vi "Add Parent.vi"(8 "error in (no error)":errorcluster, 9 "Parent ID":i32=-1, 10 "Object ID":i32=-1, 11 "Parent Child in":refnum<class "Parent Child.lvclass">) -> (0 "error out":errorcluster, 3 "Parent Child out":refnum<class "Parent Child.lvclass">)   [LabVIEW 2019, in "HierDAL Library.lvlib" / "Database.lvlib" / "Repositories.lvlib" / "Parent Child.lvclass"]
uses:
  Parent Child.lvclass
  Parent Child.lvclass/Parent Child.ctl
  Database Manager Class/Database Manager.lvclass
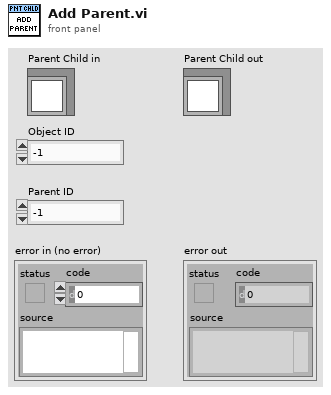
[diagram p1: front panel]
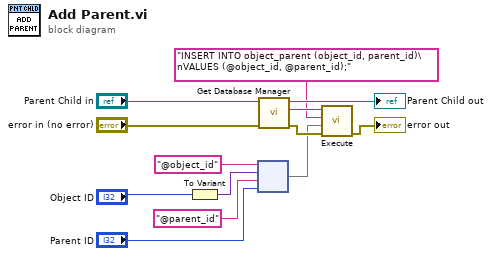
[diagram p0: block diagram]
diagram:
  n1 = To Variant(anything="Object ID") -> (Variant=w7:variant)
  n2 = node("@object_id" ("key"), w7, "@parent_id" ("key"), "Parent ID") -> (w4:map{string, variant})
  n3 = call "Get Database Manager.vi"("error in (no error)"="error in (no error)", "Parent Child in"="Parent Child in") -> ("error out"=w11:errorcluster, "Database Manager"=w10:refnum<class "Database Manager.lvclass">, "Parent Child out"=→"Parent Child out":refnum<class "Parent Child.lvclass">)  [unwired: 7 in]
  n4 = call-dynamic "Execute.vi"("error in (no error)"=w11, "Parameters"=w4, "Query"="INSERT INTO object_parent (object_id, parent_id)\nVALUES (@object_id, @parent_id);", "Database Manager in"=w10) -> ("error out"=→"error out":errorcluster)  [unwired: 5 in, 2 out]
